vi "Labview Lab 1.vi"() -> ()   [LabVIEW 2019]
uses:
  <vilib>/Instr/_visa.llb/VISA Configure Serial Port (Instr).vi
panel:
  out "read buffer":string
  in  "stop":bool
  in  "VISA resource name":refnum<visa-resource-name>
  out "Waveform Chart":dbl[][](graph)
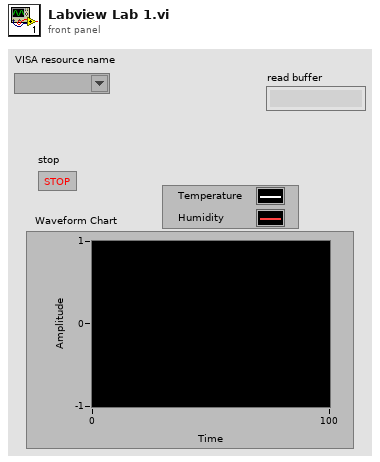
[diagram p1: front panel]
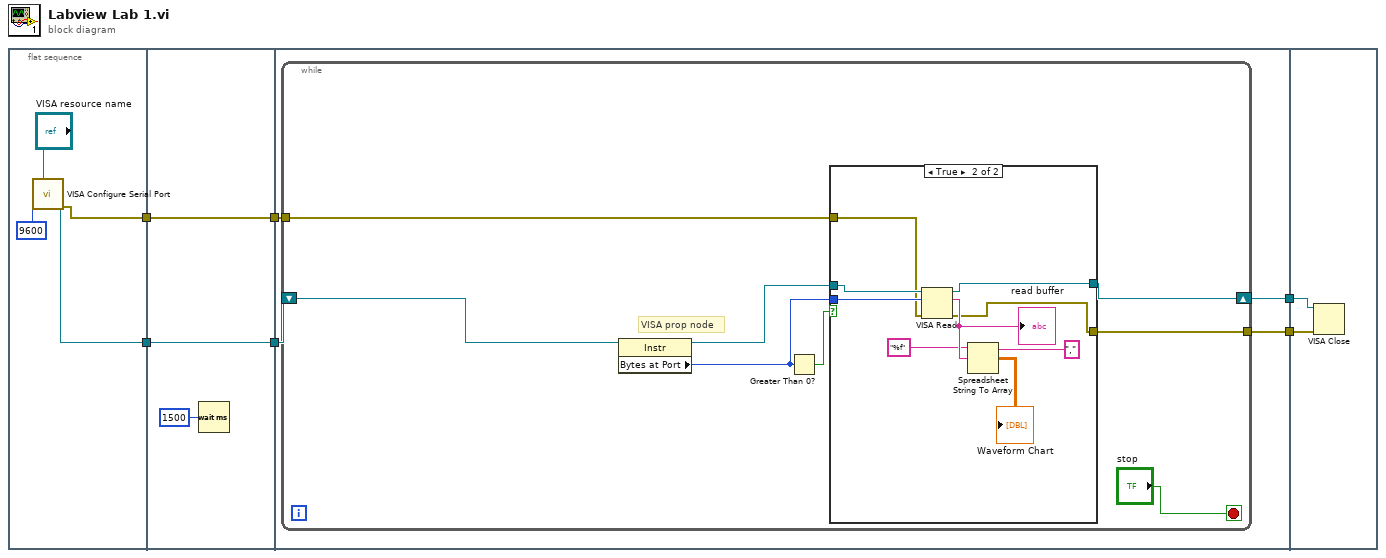
[diagram p0: block diagram]
diagram:
  n1 = flat-sequence {
    tunnel: [w10] -> w5
    tunnel: [w7] -> w2
    tunnel: [w13] -> w6
    tunnel: w5 -> [w13]
    tunnel: w2 -> [w11]
    tunnel: [w11] -> w1
    tunnel: w6 -> [w17]
    tunnel: [w16] -> w4
    tunnel: [w15] -> w3
    tunnel: w1 -> [w14]
    tunnel: w4 -> [w38]
    tunnel: w3 -> [w37]
    frame #0 {
      n2 = call-poly "VISA Configure Serial Port"("VISA resource name"="VISA resource name", "baud rate (9600)"=u32 9600) -> ("VISA resource name out"=w10:refnum<visa-resource-name>, "error out"=w7:errorcluster)  [unwired: 12 in]
    }
    frame #1 {
      n3 = Wait (ms)(milliseconds to wait=u32 1500) -> ()  [unwired: 1 out]
    }
    frame #2 {
      n4 = while {
        shift-right: [w22] -> w16
        shift-left: w17 -> [w23]
        tunnel: [w19] -> w15
        tunnel: w14 -> [w18]
        stop <- "stop" stop-if-true
        # "VISA prop node"
        n5 = property class="Instr"(reference=w23) -> (reference out=w24:refnum<visa-resource-name>, "Bytes at Port"=w21:u32)  [unwired: 1 in, 1 out]
        n6 = Greater Than 0?(x=w21) -> (x > 0?=w25:bool)
        n7 = case shown="True" w25 {
          tunnel: w24 -> [w27 w36]
          tunnel: [w27 w35] -> w22
          tunnel: w21 -> [_ w30]
          tunnel: [w26 w29] -> w19
          tunnel: w18 -> [w26 w28]
          frame False {
          }
          frame True {
            n8 = VISA Read(VISA resource name=w36, byte count=w30, error in (no error)=w28) -> (VISA resource name out=w35:refnum<visa-resource-name>, read buffer=w34:string, error out=w29:errorcluster)  [unwired: 1 out]
            "read buffer" <- w34
            n9 = Spreadsheet String To Array(delimiter (Tab)=",", format string="%f", spreadsheet string=w34) -> (array=→"Waveform Chart":dbl[][])  [unwired: 1 in]
          }
        }
      }
    }
    frame #3 {
      n10 = VISA Close(VISA resource name=w38, error in (no error)=w37) -> ()  [unwired: 1 out]
    }
  }
